vi "LHF.DB.Mongo.Util.JSONtoBSON.vi"(8 "error in (no error)":errorcluster, 10 "JSON data":string) -> (0 "error out":errorcluster, 2 "BsonValue":refnum<k24>)   [LabVIEW 2013, in "LHF.DB.Mongo.lvclass"]
uses:
  LHF.DB.Mongo.lvclass
  C:/Users/Ricardo/Desktop/Projetos/LabVIEW-MongoDB/src/Driver/MongoDB.Bson.dll
  LabVIEW-MongoDB/src/Driver/MongoDB.Bson.dll
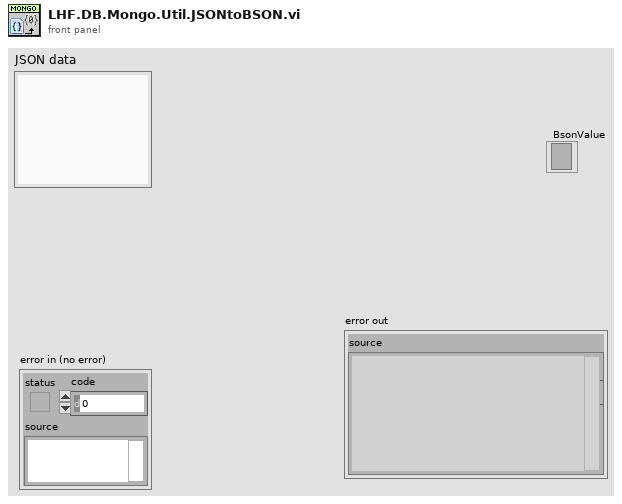
[diagram p1: front panel]
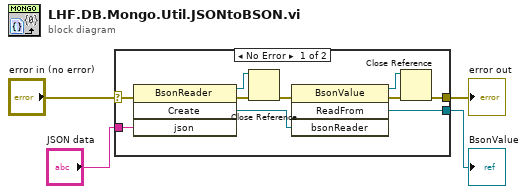
[diagram p0: block diagram]
diagram:
  n1 = case shown="No Error" "error in (no error)" {
    selector: "error in (no error)" -> [w12 w15]
    tunnel: [w6 w15] -> w3
    tunnel: [w14 _] -> w2
    tunnel: "JSON data" -> [w13 _]
    frame No Error {
      n2 = invoke class="BsonReader" method="Create"(error in=w12, "json"=w13) -> (reference out=w9:refnum<k24>, error out=w10:errorcluster, "Create"=w11:refnum<k24>)  [unwired: 2 in, 1 out]
      n3 = Close Reference(reference=w9, error in (no error)=w10) -> (error out=w8:errorcluster)
      n4 = invoke class="BsonValue" method="ReadFrom"(error in=w8, "bsonReader"=w11) -> (reference out=w5:refnum<k24>, error out=w7:errorcluster, "ReadFrom"=w14:refnum<k24>)  [unwired: 2 in, 1 out]
      n5 = Close Reference(reference=w5, error in (no error)=w7) -> (error out=w6:errorcluster)
    }
    frame Error {
    }
  }
  "error out" <- w3
  "BsonValue" <- w2
